vi "SE Session FGV.vi"(7 "Action":enum16{"Get", "Clear"}(ring), 8 "error in (no error)":errorcluster, 11 "Virtual Device Name":string="SwitchConfiguration1") -> (0 "error out":errorcluster, 3 "NISE Session (out)":T1)   [LabVIEW 2025, in "Switch Executive Controller.lvclass"]
uses:
  Switch Executive Controller.lvclass
  Switch Executive Controller.lvclass/Switch Executive Controller.ctl
  <vilib>/SwitchExecutive/nise.llb/niSE SessionRefnum.ctl
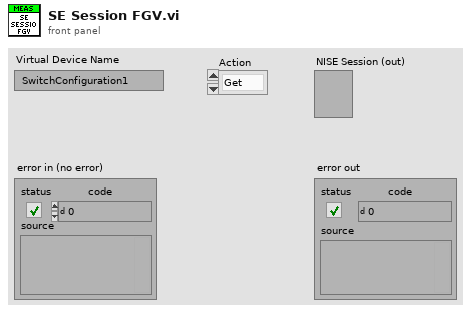
[diagram p1: front panel]
types:
  T1 = typedef "niSE SessionRefnum.ctl" = refnum<k1>
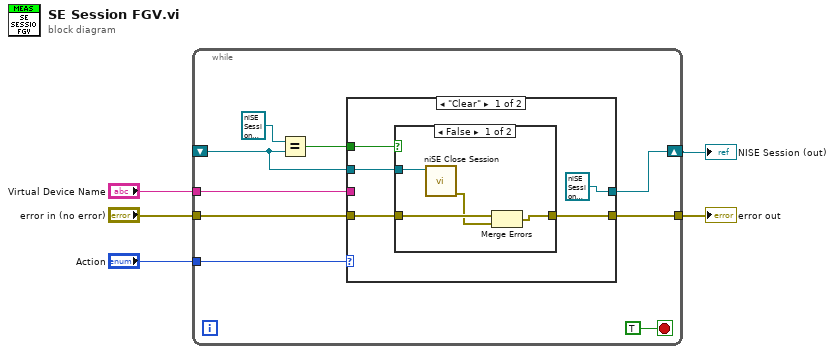
[diagram p0: block diagram]
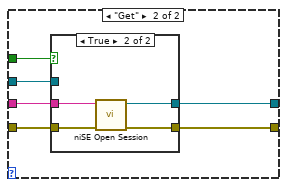
[diagram p3: hidden frame]
diagram:
  n1 = while {
    tunnel: "Virtual Device Name" -> [w14]
    tunnel: "Action" -> [w12]
    shift-right: [w11] -> w2
    shift-left: _ -> [w7]
    tunnel: [w8] -> w3
    tunnel: "error in (no error)" -> [w6]
    stop <- TRUE stop-if-true
    n2 = Equal?(x=T1 refnum ("NISE Session (out)"), y=w7) -> (x = y?=w9:bool)
    n3 = case shown="\"Clear\"" w12 {
      tunnel: w14 -> [_ w30]
      tunnel: [T1 refnum ("NISE Session (out)") w29] -> w11
      tunnel: w9 -> [w19 w28]
      tunnel: [w16 w27] -> w8
      tunnel: w7 -> [w15 w26]
      tunnel: w6 -> [w17 w25]
      frame "Clear" {
        n4 = case shown="False" w19 {
          tunnel: w17 -> [w22 w24]
          tunnel: [w21 w24] -> w16
          tunnel: w15 -> [w23 _]
          frame False {
            n5 = call <vilib>:"niSE Close Session.vi"("NISE Session (in)"=w23) -> ("error out"=w20:errorcluster)  [unwired: 6 in]
            n6 = Merge Errors(w22, w20) -> (w21:errorcluster)
          }
          frame True {
          }
        }
      }
      frame "Get" {
        n7 = case shown="True" w28 {
          tunnel: w30 -> [_ w36]
          tunnel: [w32 w35] -> w29
          tunnel: [w31 w34] -> w27
          tunnel: w26 -> [w32 _]
          tunnel: w25 -> [w31 w33]
          frame False {
          }
          frame True {
            n8 = call <vilib>:"niSE Open Session.vi"("error in (no error)"=w33, "Virtual Device Name (SwitchConfiguration1)"=w36) -> ("error out"=w34:errorcluster, "NISE Session (out)"=w35:T1)  [unwired: 4 in]
          }
        }
      }
    }
  }
  "error out" <- w3
  "NISE Session (out)" <- w2
